vi "UI_Gear_Unit_Test2.vi"() -> ()   [LabVIEW 2014]
panel:
  out "冷却装置工作状态S":dbl(graph)
  out "齿轮箱油站调试状态":bool
  in  "退出":bool
  in  "开始调试":bool
  in  "齿轮子系统供油流量过低":bool caption="供油流量过低"
  in  "齿轮子系统供油压力过低":bool caption="供油压力过低"
  in  "齿轮子系统2号油泵故障":bool caption="2号油泵故障"
  in  "齿轮子系统1号油泵故障":bool caption="1号油泵故障"
  in  "齿轮子系统回油过滤器压差过高":bool caption="回油过滤器压差过高"
  in  "齿轮子系统循环回路过滤器压差过高":bool caption="循环回路过滤器压差过高"
  in  "齿轮子系统供油过滤器压差过高":bool caption="供油过滤器压差过高"
  in  "齿轮子系统供油油温过高":bool caption="供油油温过高"
  in  "齿轮子系统油箱液位过低":bool caption="油箱液位过低"
  in  "齿轮子系统油箱液位过高":bool caption="油箱液位过高"
  in  "齿轮子系统冷却装置异常":bool caption="冷却装置异常"
  in  "齿轮子系统加热装置异常":bool caption="加热装置异常"
  out "供油油温":dbl(graph)
  out "油箱液位":dbl(graph)
  out "过滤器压差":dbl(graph)
  out "供油压力":dbl(graph)
  out "油箱润滑油液位":dbl(graph)
  out "润滑油流量":dbl(graph)
  out "油箱温度":dbl(graph)
  # "齿轮箱油站独立调试"
  # "监测参数"
  # "报警信息"
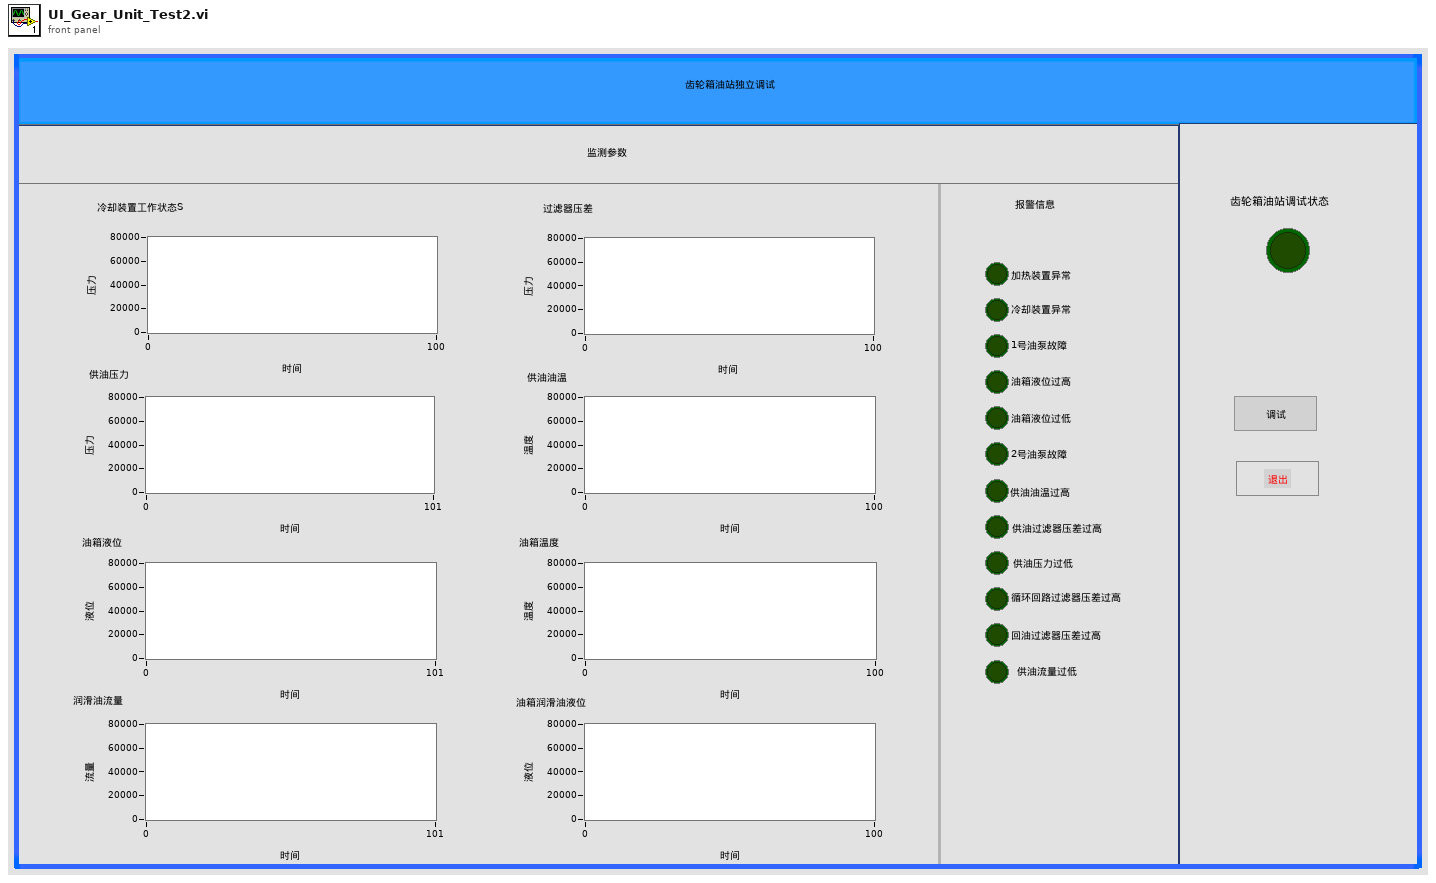
[diagram p1: front panel]
types:
  T1 = cluster{"润滑油流量":u16, "油箱润滑油液位":u16, "油箱温度":u16, "冷却装置工作状态":u16, "供油压力":u16, "过滤器压差":u16, "油箱液位":u16, "供油油温":u16, "齿轮箱轴承温度":u16, "齿轮箱高速端输出转速":u16, "齿轮子系统状态字":cluster{"加热装置异常报警":bool, "冷却装置异常报警":bool, "油箱液位过低报警":bool, "供油油温过高报警":bool, "循环回路过滤器压差过高报警":bool, "1号油泵故障报警":bool, "2号油泵故障报警":bool, "供油压力过低报警":bool, "供油流量过低报警":bool, "轴承温度异常报警":bool, "油箱液位过高报警":bool, "回油过滤器压差过高报警":bool, "供油过滤器压差过高报警":bool}}
  T2 = cluster{"时间":timestamp, "陪试轴承润滑单元出油温度1":sgl[], "陪试轴承润滑单元出油温度2":sgl[], "轴承外圈温度":sgl[], "出油温度":sgl[], "摩擦力1":sgl[], "摩擦力2":sgl[], "径向油缸力":sgl[], "轴向油缸力":sgl[], "转速":sgl[]}
  T3 = cluster{"加热装置异常报警":bool, "冷却装置异常报警":bool, "油箱液位过低报警":bool, "供油油温过高报警":bool, "循环回路过滤器压差过高报警":bool, "1号油泵故障报警":bool, "2号油泵故障报警":bool, "供油压力过低报警":bool, "供油流量过低报警":bool, "轴承温度异常报警":bool, "油箱液位过高报警":bool, "回油过滤器压差过高报警":bool, "供油过滤器压差过高报警":bool}
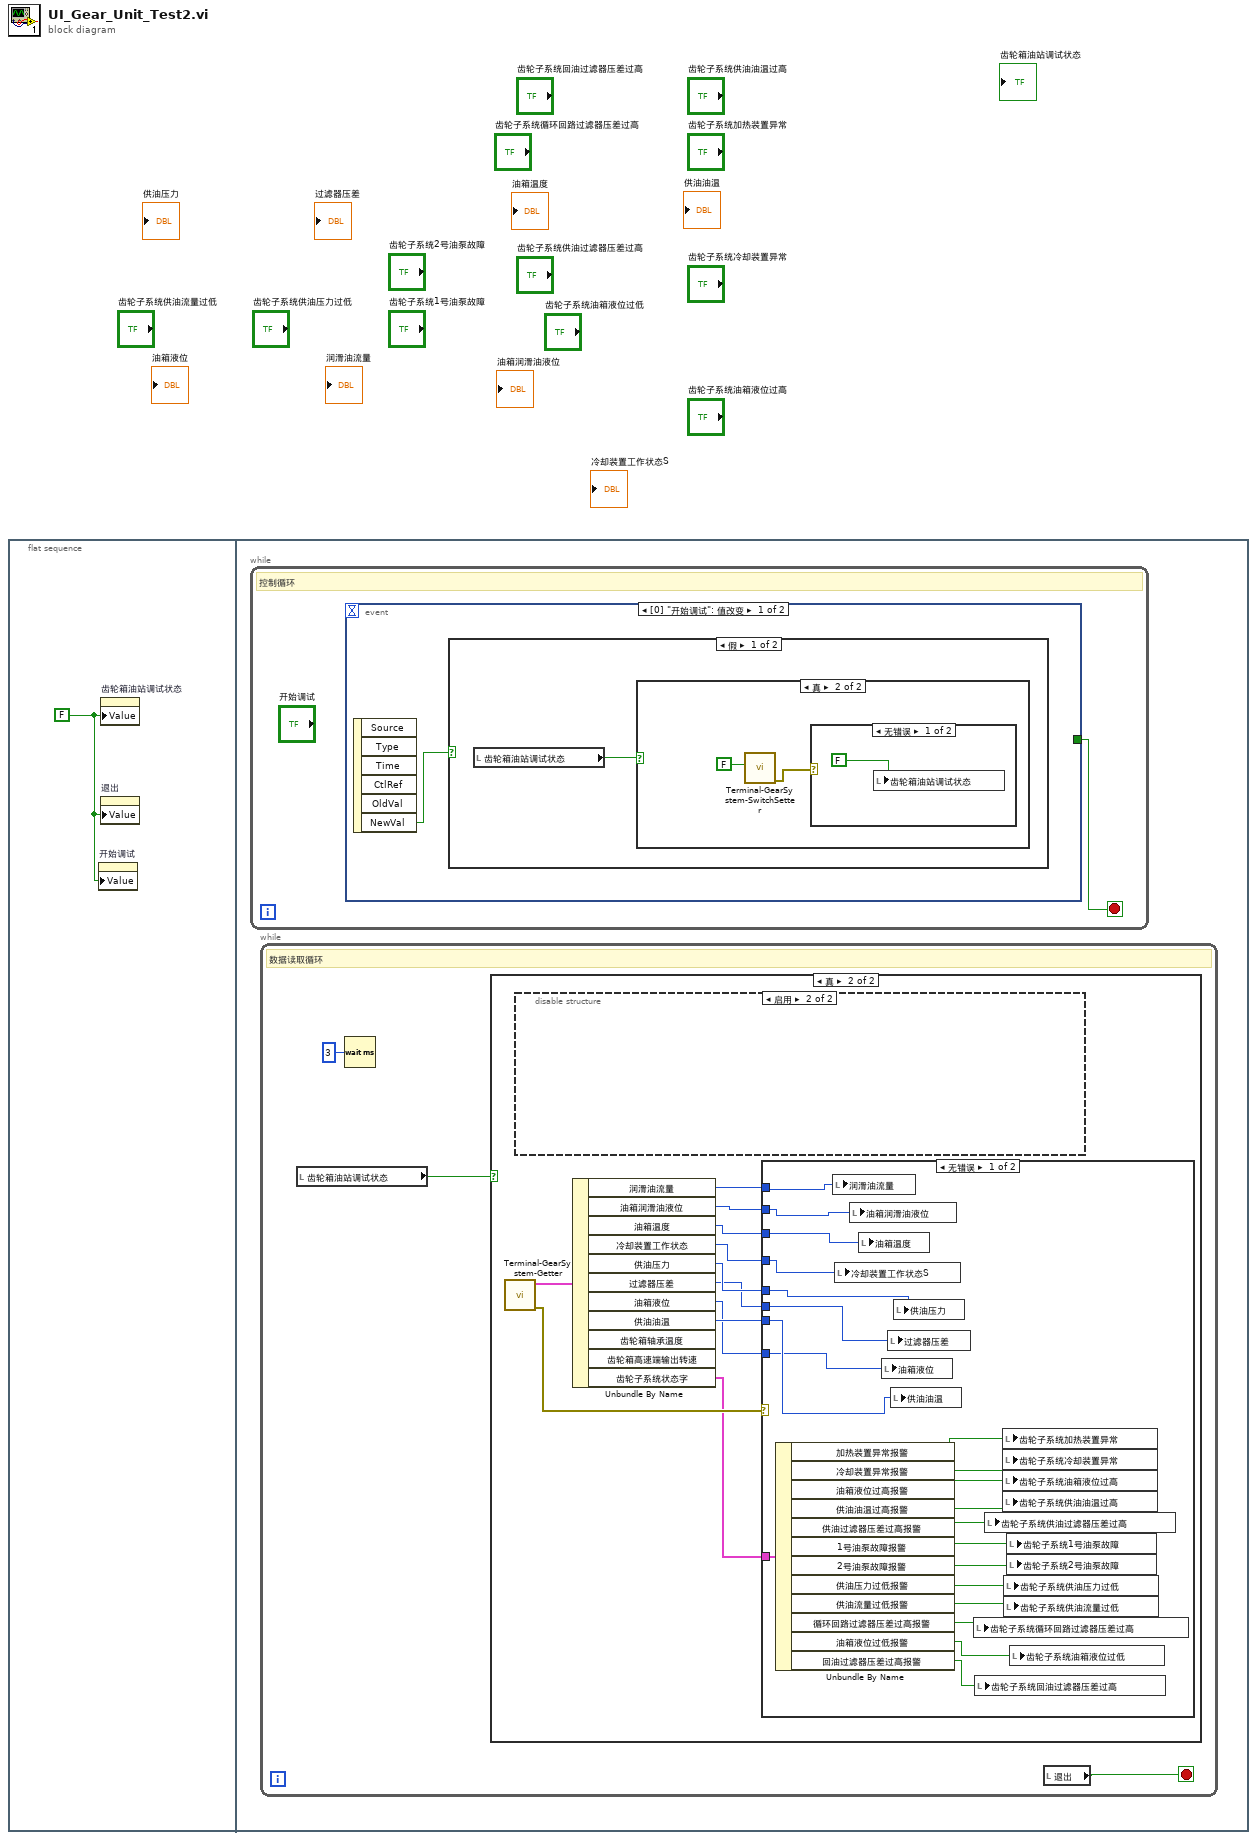
[diagram p0: block diagram]
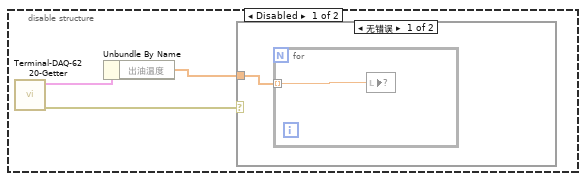
[diagram p3: hidden frame]
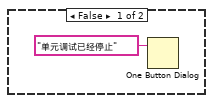
[diagram p6: hidden frame]
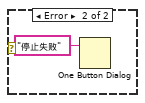
[diagram p7: hidden frame]
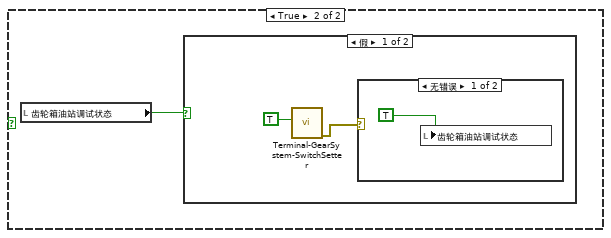
[diagram p8: hidden frame]
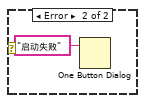
[diagram p9: hidden frame]
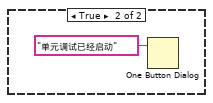
[diagram p10: hidden frame]
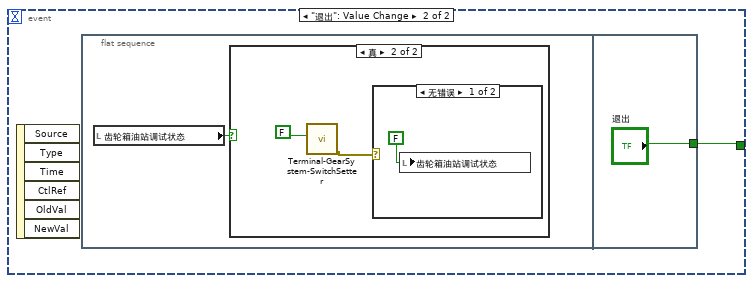
[diagram p11: hidden frame]
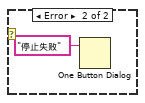
[diagram p13: hidden frame]
diagram:
  n1 = flat-sequence {
    frame #0 {
      w1 = FALSE ("齿轮箱油站调试状态")
      n2 = property on="开始调试" class="Bool (严格)"("Value"=w1) -> ()  [unwired: 2 in, 2 out]
      n3 = property on="齿轮箱油站调试状态" class="Bool (严格)"("Value"=w1) -> ()  [unwired: 2 in, 2 out]
      n4 = property on="退出" class="Bool (严格)"("Value"=w1) -> ()  [unwired: 2 in, 2 out]
    }
    frame #1 {
      n5 = while {
        stop <- w42 stop-if-true
        # "控制循环"
        n6 = event shown="[0] \"开始调试\": 值改变" {
          selector: _ -> [_ _]
          dyn-events: _ -> [_ _]
          timeout: _ -> [_ _]
          tunnel: [_ w56] -> w42
          event "开始调试": Value Change {
            n7 = event-data() -> ("NewVal"=w43:bool)  [unwired: 1 in, 5 out]
            n8 = case shown="假" w43 {
              frame False {
                n9 = local read "齿轮箱油站调试状态"() -> (w44:bool)
                n10 = case shown="真" w44 {
                  frame False {
                    n11 = One Button Dialog(message="单元调试已经停止" ("消息")) -> ()  [unwired: 1 in, 1 out]
                  }
                  frame True {
                    n12 = call "Terminal-GearSystem-SwitchSetter.vi"("启停"=FALSE) -> ("error out"=w46:errorcluster)  [unwired: 10 in]
                    n13 = case shown="无错误" w46 {
                      frame No Error {
                        n14 = local write "齿轮箱油站调试状态"(FALSE) -> ()
                      }
                      frame Error {
                        n15 = One Button Dialog(message="停止失败" ("消息")) -> ()  [unwired: 1 in, 1 out]
                      }
                    }
                  }
                }
              }
              frame True {
                n16 = local read "齿轮箱油站调试状态"() -> (w50:bool)
                n17 = case shown="假" w50 {
                  frame False {
                    n18 = call "Terminal-GearSystem-SwitchSetter.vi"("启停"=TRUE) -> ("error out"=w51:errorcluster)  [unwired: 10 in]
                    n19 = case shown="无错误" w51 {
                      frame No Error {
                        n20 = local write "齿轮箱油站调试状态"(TRUE) -> ()
                      }
                      frame Error {
                        n21 = One Button Dialog(message="启动失败" ("消息")) -> ()  [unwired: 1 in, 1 out]
                      }
                    }
                  }
                  frame True {
                    n22 = One Button Dialog(message="单元调试已经启动" ("消息")) -> ()  [unwired: 1 in, 1 out]
                  }
                }
              }
            }
          }
          event "退出": Value Change {
            n23 = event-data() -> ()  [unwired: 1 in, 6 out]
            n24 = flat-sequence {
              tunnel: ["退出"] -> w56
              frame #0 {
                n25 = local read "齿轮箱油站调试状态"() -> (w57:bool)
                n26 = case shown="真" w57 {
                  frame False {
                  }
                  frame True {
                    n27 = call "Terminal-GearSystem-SwitchSetter.vi"("启停"=FALSE) -> ("error out"=w59:errorcluster)  [unwired: 10 in]
                    n28 = case shown="无错误" w59 {
                      frame No Error {
                        n29 = local write "齿轮箱油站调试状态"(FALSE) -> ()
                      }
                      frame Error {
                        n30 = One Button Dialog(message="停止失败" ("消息")) -> ()  [unwired: 1 in, 1 out]
                      }
                    }
                  }
                }
              }
              frame #1 {
              }
            }
          }
        }
      }
      n31 = while {
        stop <- w3 stop-if-true
        # "数据读取循环"
        n32 = local read "齿轮箱油站调试状态"() -> (w4:bool)
        n33 = Wait (ms)(milliseconds to wait=u32 3 ("等待时间（毫秒）")) -> ()  [unwired: 1 out]
        n34 = case shown="真" w4 {
          frame False {
          }
          frame True {
            n35 = call "Terminal-GearSystem-Getter.vi"() -> ("error out"=w15:errorcluster, "设备信息"=w5:T1)  [unwired: 10 in]
            n36 = disable-structure shown="启用" {
              frame Disabled {
                n37 = call "Terminal-DAQ-6220-Getter.vi"() -> ("error out"=w18:errorcluster, "6220"=w17:T2)  [unwired: 10 in]
                n38 = Unbundle By Name(w17) -> ("出油温度"=w16:sgl[])
                n39 = case shown="无错误" w18 {
                  tunnel: w16 -> [w19 _]
                  frame No Error {
                    n40 = for {
                      tunnel: w19 -> [w20] mode=indexing
                      n41 = local write item#-1(w20) -> ()
                    }
                  }
                  frame Error {
                  }
                }
              }
              frame Enabled {
              }
            }
            n42 = Unbundle By Name(w5) -> ("润滑油流量"=w13:u16, "油箱润滑油液位"=w12:u16, "油箱温度"=w11:u16, "冷却装置工作状态"=w10:u16, "供油压力"=w9:u16, "过滤器压差"=w8:u16, "油箱液位"=w6:u16, "供油油温"=w7:u16, "齿轮子系统状态字"=w14:T3)  [unwired: 2 out]
            n43 = case shown="无错误" w15 {
              tunnel: w14 -> [w27 _]
              tunnel: w13 -> [w24 _]
              tunnel: w12 -> [w23 _]
              tunnel: w11 -> [w41 _]
              tunnel: w10 -> [w21 _]
              tunnel: w9 -> [w40 _]
              tunnel: w8 -> [w39 _]
              tunnel: w7 -> [w38 _]
              tunnel: w6 -> [w22 _]
              frame No Error {
                n44 = Unbundle By Name(w27) -> ("加热装置异常报警"=w37:bool, "冷却装置异常报警"=w36:bool, "油箱液位过高报警"=w35:bool, "供油油温过高报警"=w34:bool, "供油过滤器压差过高报警"=w33:bool, "1号油泵故障报警"=w32:bool, "2号油泵故障报警"=w31:bool, "供油压力过低报警"=w30:bool, "供油流量过低报警"=w29:bool, "循环回路过滤器压差过高报警"=w28:bool, "油箱液位过低报警"=w26:bool, "回油过滤器压差过高报警"=w25:bool)
                n45 = local write "润滑油流量"(w24) -> ()
                n46 = local write "冷却装置工作状态S"(w21) -> ()
                n47 = local write "油箱润滑油液位"(w23) -> ()
                n48 = local write "油箱温度"(w41) -> ()
                n49 = local write "油箱液位"(w22) -> ()
                n50 = local write "过滤器压差"(w39) -> ()
                n51 = local write "供油油温"(w38) -> ()
                n52 = local write "供油压力"(w40) -> ()
                n53 = local write "齿轮子系统循环回路过滤器压差过高"(w28) -> ()
                n54 = local write "齿轮子系统回油过滤器压差过高"(w25) -> ()
                n55 = local write "齿轮子系统供油过滤器压差过高"(w33) -> ()
                n56 = local write "齿轮子系统加热装置异常"(w37) -> ()
                n57 = local write "齿轮子系统冷却装置异常"(w36) -> ()
                n58 = local write "齿轮子系统油箱液位过高"(w35) -> ()
                n59 = local write "齿轮子系统供油油温过高"(w34) -> ()
                n60 = local write "齿轮子系统供油压力过低"(w30) -> ()
                n61 = local write "齿轮子系统供油流量过低"(w29) -> ()
                n62 = local write "齿轮子系统1号油泵故障"(w32) -> ()
                n63 = local write "齿轮子系统2号油泵故障"(w31) -> ()
                n64 = local write "齿轮子系统油箱液位过低"(w26) -> ()
              }
              frame Error {
              }
            }
          }
        }
        n65 = local read "退出"() -> (w3:bool)
      }
    }
  }
